vi "Right Motor Angle Loop (SubVI).vi"   [LabVIEW 2015]
uses:
  Right Variables.vi
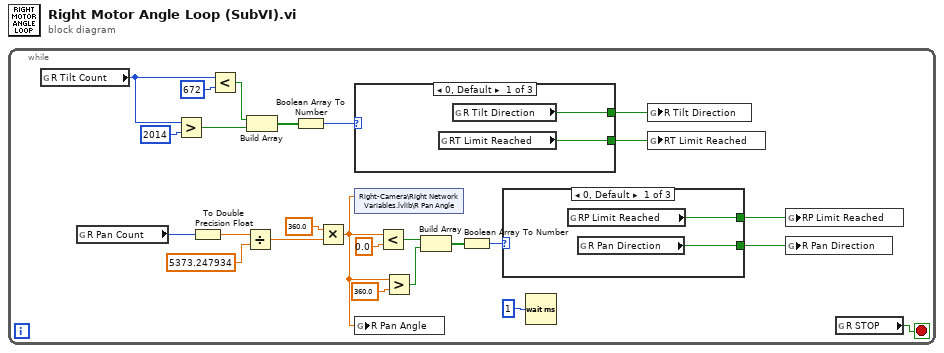
[diagram p0: block diagram]
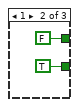
[diagram p2: hidden frame]
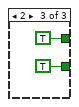
[diagram p3: hidden frame]
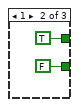
[diagram p4: hidden frame]
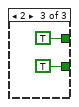
[diagram p5: hidden frame]
diagram:
  n1 = while {
    stop <- w19 stop-if-true
    n2 = global read "Right Variables.vi" "R Tilt Count"() -> (w12:i32)
    n3 = global read "Right Variables.vi" "R Pan Count"() -> (w20:i32)
    n4 = Greater?(x=w12, y=2014 ("lower limit")) -> (0:w10:bool)
    n5 = To Double Precision Float(number=w20) -> (double precision float=w23:dbl)
    n6 = Less?(x=w12, y=672 ("upper limit")) -> (x < y?=w11:bool)
    n7 = Divide(x=w23, y=5373.247934) -> (x/y=w25:dbl)
    n8 = Build Array(w11, w10) -> (w9:bool[])
    n9 = Boolean Array To Number(Boolean array=w9) -> (number=w8:u32)
    n10 = Multiply(x=360.0, y=w25) -> (x*y=w15:dbl)
    n11 = case shown="0, Default" w8 {
      tunnel: [w26 TRUE TRUE] -> w7
      tunnel: [w27 FALSE TRUE] -> w1
      frame 0, Default {
        n12 = global read "Right Variables.vi" "RT Limit Reached"() -> (w26:bool)
        n13 = global read "Right Variables.vi" "R Tilt Direction"() -> (w27:bool)
      }
      frame 1 {
      }
      frame 2 {
      }
    }
    n14 = shared-variable "Right-Camera\\Right Network Variables.lvlib\\R Pan Angle"(w15) -> ()  [unwired: 1 in, 1 out]
    n15 = global write "Right Variables.vi" "R Pan Angle"(w15) -> ()
    n16 = Less?(x=w15, y=0.0) -> (x < y?=w5:bool)
    n17 = Greater?(x=w15, y=360.0) -> (0:w4:bool)
    n18 = Build Array(w5, w4) -> (w6:bool[])
    n19 = Boolean Array To Number(Boolean array=w6) -> (number=w3:u32)
    n20 = case shown="0, Default" w3 {
      tunnel: [w33 FALSE TRUE] -> w16
      tunnel: [w32 TRUE TRUE] -> w2
      frame 0, Default {
        n21 = global read "Right Variables.vi" "RP Limit Reached"() -> (w32:bool)
        n22 = global read "Right Variables.vi" "R Pan Direction"() -> (w33:bool)
      }
      frame 1 {
      }
      frame 2 {
      }
    }
    n23 = Wait (ms)(milliseconds to wait=u32 1) -> ()  [unwired: 1 out]
    n24 = global write "Right Variables.vi" "R Tilt Direction"(w1) -> ()
    n25 = global write "Right Variables.vi" "RT Limit Reached"(w7) -> ()
    n26 = global write "Right Variables.vi" "RP Limit Reached"(w2) -> ()
    n27 = global write "Right Variables.vi" "R Pan Direction"(w16) -> ()
    n28 = global read "Right Variables.vi" "R STOP"() -> (w19:bool)
  }
